vi "multimeter.vi"() -> ()   [LabVIEW 2018]
panel:
  out "Digital Indicator":dbl
  out "R":bool
  out "I":bool
  out "V":bool
  in  "I selector":u16(ring) items=["on", "off"]
  in  "V selector":u16(ring) items=["on"=1, "off"=0]
  in  "R selector":u16(ring) items=["on", "off"]
  in  "resistance":bool
  in  "current":bool
  in  "voltage":bool
  out "Meter":dbl(knob) scale=0.0..10.0
  in  "Kohms":dbl(slide) scale=0.0..10.0
  in  "ohm":dbl(slide) scale=0.0..10.0
  in  "A":dbl(knob) scale=0.0..10.0
  in  "mA":dbl(knob) scale=0.0..10.0
  in  "uA":dbl(knob) scale=0.0..10.0
  in  "V":dbl(knob) scale=0.0..10.0
  in  "mV":dbl(knob) scale=0.0..10.0
  in  "uV":dbl(knob) scale=0.0..10.0
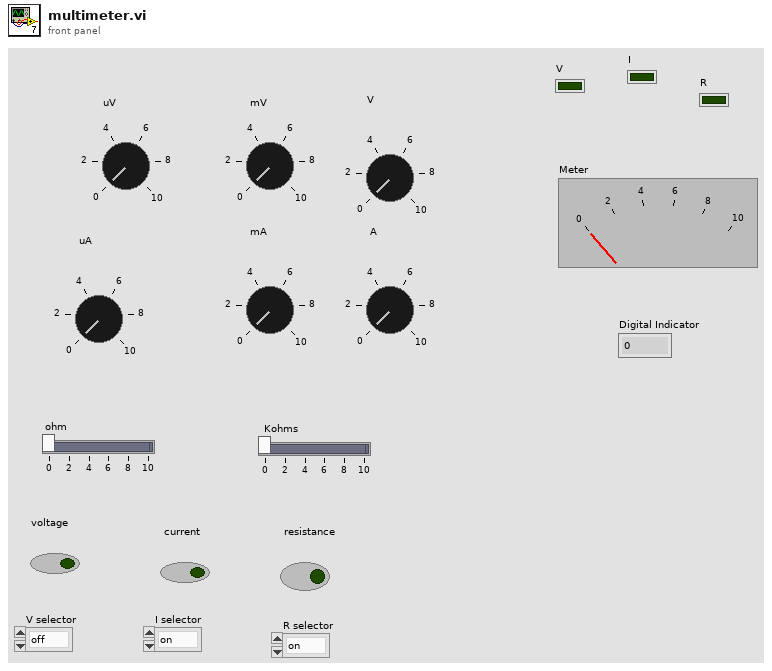
[diagram p1: front panel]
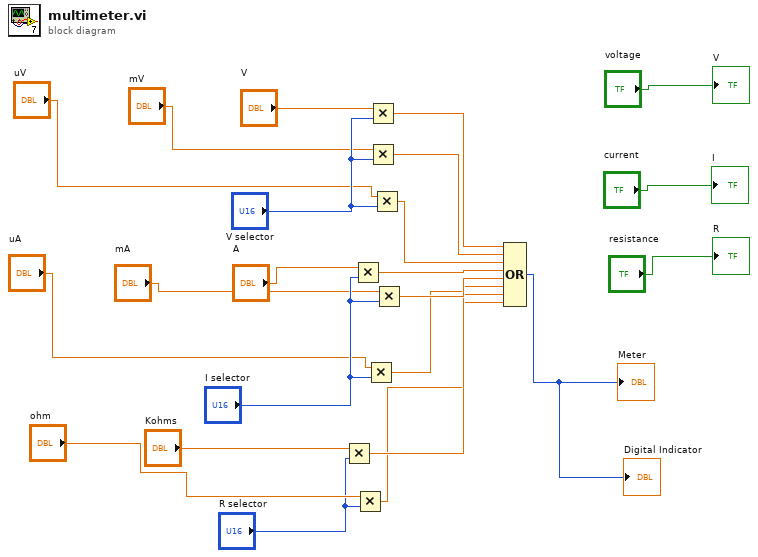
[diagram p0: block diagram]
diagram:
  n1 = Multiply(x="Kohms", y="R selector") -> (x*y=w6:dbl)
  n2 = Multiply(x="A", y="I selector") -> (x*y=w9:dbl)
  n3 = Multiply(x="ohm", y="R selector") -> (x*y=w5:dbl)
  n4 = Multiply(x="uA", y="I selector") -> (x*y=w7:dbl)
  n5 = Multiply(x="V", y="V selector") -> (x*y=w12:dbl)
  n6 = Multiply(x="mV", y="V selector") -> (x*y=w11:dbl)
  n7 = Multiply(x="uV", y="V selector") -> (x*y=w10:dbl)
  n8 = Multiply(x="mA", y="I selector") -> (x*y=w8:dbl)
  n9 = Compound Arithmetic op=OR(w12, w11, w10, w9, w8, w7, w6, w5) -> (→"Meter" →"Digital Indicator":i32)
  "V" <- "voltage"
  "I" <- "current"
  "R" <- "resistance"
